vi "PRIME Telescope Home Focus.vi"(8 "error in (no error)":errorcluster, 11 "connection ID":refnum<k5>) -> (0 "error out":errorcluster)   [LabVIEW 2021, in "PRIME Telescope.lvclass"]
uses:
  PRIME Telescope.lvclass
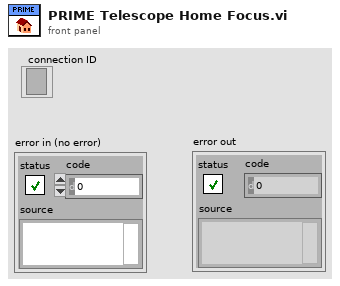
[diagram p1: front panel]
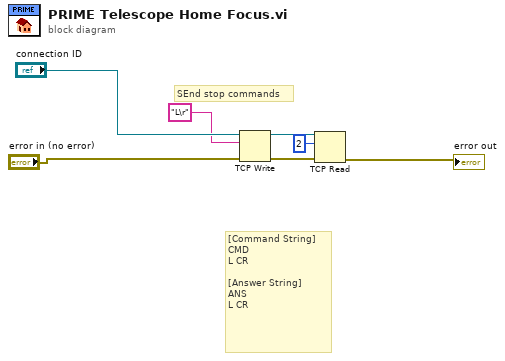
[diagram p0: block diagram]
diagram:
  # "[Command String]\nCMD\t\nL\tCR\n\t\n[Answer String]\nANS\t\nL\tCR"
  # "SEnd stop commands"
  n1 = TCP Write(connection ID="connection ID", data in="L\r", error in (no error)="error in (no error)") -> (connection ID out=w6:refnum<k5>, error out=w7:errorcluster)  [unwired: 1 in, 1 out]
  n2 = TCP Read(connection ID=w6, bytes to read=2, error in (no error)=w7) -> (error out=→"error out":errorcluster)  [unwired: 2 in, 2 out]
